vi "Drive Problem Fix.vi"(1 "Drive Info Modified":T1, 2 "Drive Info Original":T1) -> (0 "Drive Info Fixed":T1)   [LabVIEW 2013]
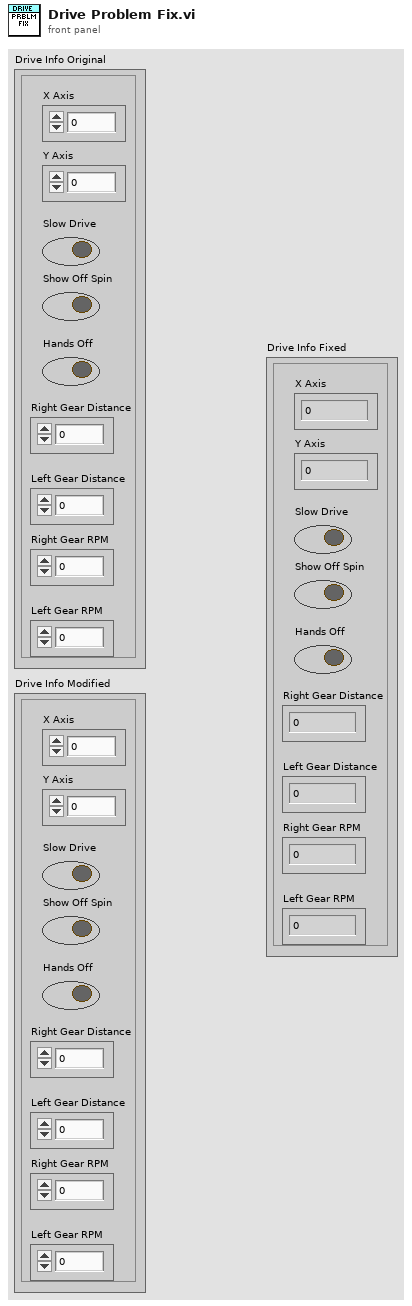
[diagram p1: front panel]
types:
  T1 = cluster{"X Axis":dbl, "Y Axis":dbl, "Slow Drive":bool, "Show Off Spin":bool, "Hands Off":bool, "Right Gear Distance":dbl, "Left Gear Distance ":dbl, "Right Gear RPM":dbl, "Left Gear RPM":dbl}
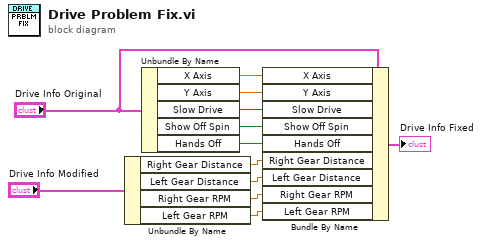
[diagram p0: block diagram]
diagram:
  n1 = Unbundle By Name("Drive Info Modified") -> ("Right Gear Distance"=w4:dbl, "Left Gear Distance"=w3:dbl, "Right Gear RPM"=w2:dbl, "Left Gear RPM"=w1:dbl)
  n2 = Unbundle By Name("Drive Info Original") -> ("X Axis"=w9:dbl, "Y Axis"=w8:dbl, "Slow Drive"=w7:bool, "Show Off Spin"=w6:bool, "Hands Off"=w5:bool)
  n3 = Bundle By Name(cluster="Drive Info Original", "X Axis"=w9, "Y Axis"=w8, "Slow Drive"=w7, "Show Off Spin"=w6, "Hands Off"=w5, "Right Gear Distance"=w4, "Left Gear Distance"=w3, "Right Gear RPM"=w2, "Left Gear RPM"=w1) -> (→"Drive Info Fixed":T1)
